vi "4155C Get Threshold Voltage.vi"(8 "Input I":dbl[](array[numeric]) format="%.2f", 9 "VG":dbl[](array[numeric]) format="%.2f", 11 "Threshold ratio":dbl=3.0 format="%.2f") -> (2 "Threshold Voltage":string)   [LabVIEW 2016]
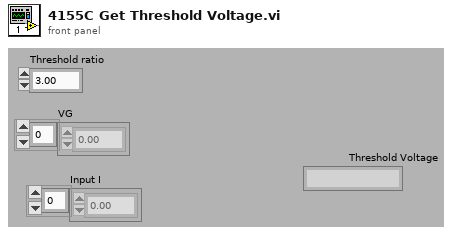
[diagram p1: front panel]
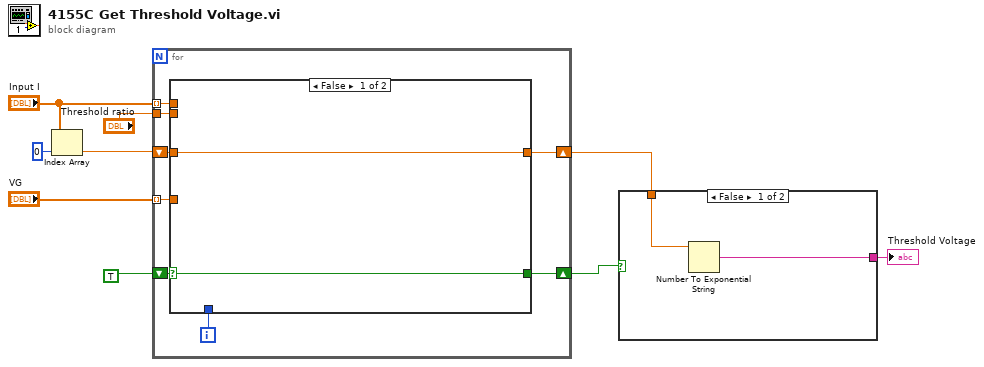
[diagram p0: block diagram]
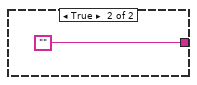
[diagram p2: hidden frame]
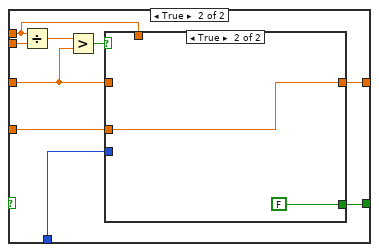
[diagram p3: hidden frame]
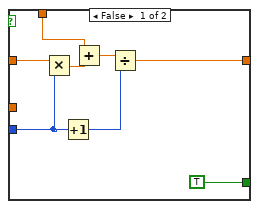
[diagram p4: hidden frame]
diagram:
  n1 = Index Array(array="Input I", index=0 ("Index")) -> (element=w7:dbl)
  n2 = for {
    tunnel: "Input I" -> [w17] mode=indexing
    shift-right: [w13] -> w2
    shift-left: w7 -> [w15]
    tunnel: "Threshold ratio" -> [w16]
    shift-right: [w12] -> w3
    shift-left: TRUE -> [w14]
    tunnel: "VG" -> [w11] mode=indexing
    i -> [w10]
    n3 = case shown="False" w14 {
      selector: w14 -> [w18 _]
      tunnel: w17 -> [_ w20]
      tunnel: w16 -> [_ w28]
      tunnel: w15 -> [w19 w23]
      tunnel: [w19 w24] -> w13
      tunnel: [w18 w26] -> w12
      tunnel: w11 -> [_ w25]
      tunnel: w10 -> [_ w22]
      frame False {
      }
      frame True {
        n4 = Divide(x=w20, y=w28) -> (x/y=w21:dbl)
        n5 = Greater?(x=w21, y=w23) -> (0:w27:bool)
        n6 = case shown="True" w27 {
          tunnel: [TRUE FALSE] -> w26
          tunnel: w25 -> [_ w37]
          tunnel: [w29 w37] -> w24
          tunnel: w23 -> [w35 _]
          tunnel: w22 -> [w31 _]
          tunnel: w20 -> [w34 _]
          frame False {
            n7 = Multiply(x=w35, y=w31) -> (x*y=w33:dbl)
            n8 = Increment(x=w31) -> (x+1=w30:i32)
            n9 = Add(x=w34, y=w33) -> (x+y=w32:dbl)
            n10 = Divide(x=w32, y=w30) -> (x/y=w29:dbl)
          }
          frame True {
          }
        }
      }
    }
  }
  n11 = case shown="False" w3 {
    tunnel: w2 -> [w40 _]
    tunnel: [w39 ""] -> w1
    frame False {
      n12 = Number To Exponential String(number=w40) -> (E-format string=w39:string)  [unwired: 3 in]
    }
    frame True {
    }
  }
  "Threshold Voltage" <- w1
